vi "mod_Modulate AM (DSB).vi"(0 "message signal":waveform(dbl)={"t0"=timestamp(0 s since 1904-01-01), "dt"=0.0, "Y"=[]}, 5 "modulation index":dbl=1.0 format="%.2f", 9 "peak message amplitude":dbl=1.0, 11 "error in (no error)":errorcluster, 12 "suppress carrier ?":bool) -> (4 "AM modulated waveform":cluster{"t0":dbl, "dt":dbl, "Y":cdb[]} {"Y" format="%.2f"; "dt" format="%.2f"; "t0" format="%.2f"}, 15 "error out":errorcluster)   [LabVIEW 2020, in "niAMT.lvlib"]
doc: "Performs a double sideband (DSB) amplitude modulation on an RF carrier wave according to a baseband information signal which is input to the <B>message signal</B> control. It returns the complex envelope of the AM modulated signal in the <B>AM modulated waveform</B> indicator. \n\nThis VI is used with simulated data and operates independently of your hardware settings."
uses:
  <vilib>/addons/Modulation/niAMT.lvlib
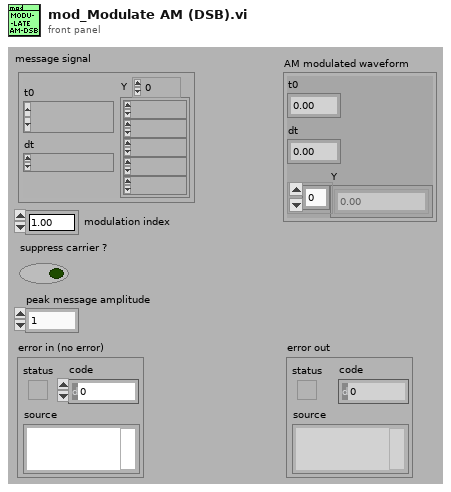
[diagram p1: front panel]
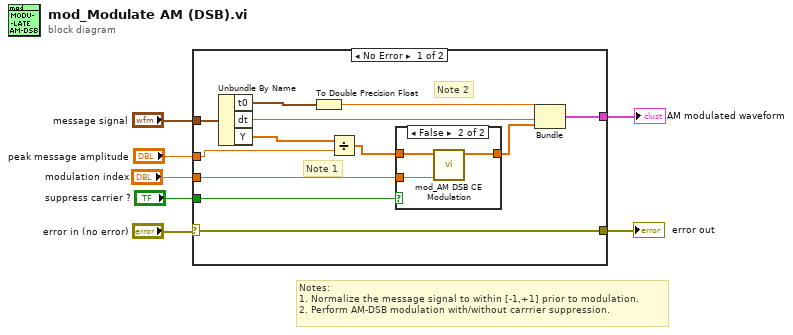
[diagram p0: block diagram]
diagram:
  # "Notes:\n1. Normalize the message signal to within [-1,+1] prior to modulation.\n2. Perform AM-DSB modulation with/without carrrier suppression."
  n1 = case shown="No Error" "error in (no error)" {
    selector: "error in (no error)" -> [w19 w24]
    tunnel: [w19 w24] -> w7
    tunnel: "modulation index" -> [w17 _]
    tunnel: "message signal" -> [w18 _]
    tunnel: [w14 _] -> w3
    tunnel: "suppress carrier ?" -> [w11 _]
    tunnel: "peak message amplitude" -> [w9 _]
    frame No Error {
      # "Note 2"
      # "Note 1"
      n2 = Unbundle By Name(w18) -> ("t0"=w13:timestamp, "dt"=w15:dbl, "Y"=w10:dbl[])
      n3 = To Double Precision Float(number=w13) -> (double precision float=w16:dbl)
      n4 = Divide(x=w10, y=w9) -> (x/y=w8:dbl[])
      n5 = case shown="False" w11 {
        tunnel: w8 -> [w20 w21]
        tunnel: w17 -> [_ w23]
        tunnel: [w20 w22] -> w12
        frame True {
        }
        frame False {
          n6 = call <vilib>:"mod_AM DSB CE Modulation.vi"("ka"=w23, "x"=w21) -> ("AM DSB CE"=w22:cdb[])  [unwired: 1 in, 8 out]
        }
      }
      n7 = Bundle(w16, "dt"=w15, "AM DSB CE"=w12) -> (w14:cluster{dbl, "dt":dbl, "AM DSB CE":cdb[]})  [unwired: 1 out]
    }
    frame Error {
    }
  }
  "error out" <- w7
  "AM modulated waveform" <- w3
